vi "Init.vi"(8 "error in (no error)":errorcluster, 10 "IConfigure":refnum<class "IConfigure.lvclass">, 11 "Camera Imaqdx in":refnum<class "Camera Imaqdx.lvclass">=refnum) -> (0 "error out":errorcluster, 3 "Camera Imaqdx out":refnum<class "Camera Imaqdx.lvclass">)   [LabVIEW 2023]
uses:
  Configuration/Camera Imaqdx CFG.lvclass
  Interfaces/IConfigure/IConfigure.lvclass
  Camera Imaqdx.lvclass
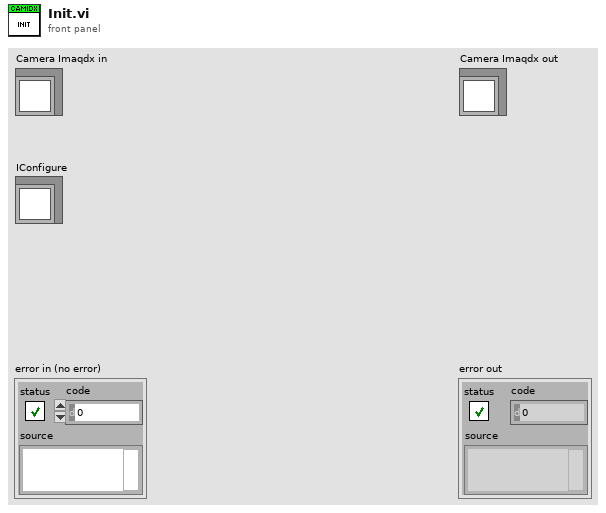
[diagram p1: front panel]
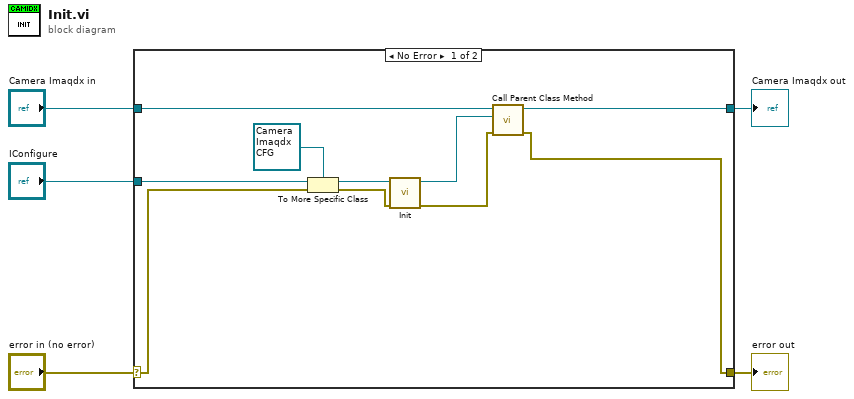
[diagram p0: block diagram]
diagram:
  n1 = case shown="No Error" "error in (no error)" {
    selector: "error in (no error)" -> [w6 w17]
    tunnel: [w8 w17] -> w4
    tunnel: [w12 w16] -> w2
    tunnel: "Camera Imaqdx in" -> [w7 w16]
    tunnel: "IConfigure" -> [w11 _]
    frame No Error {
      n2 = To More Specific Class(target class=refnum<class "Camera Imaqdx CFG.lvclass"> refnum ("Cameras.lvlib:Camera Config Imaqdx.lvclass"), reference=w11, error in=w6) -> (specific class reference=w14:refnum<class "Camera Imaqdx CFG.lvclass">, error out=w13:errorcluster)
      n3 = call-dynamic "Init.vi"("error in"=w13, "Camera Config Imaqdx in"=w14) -> ("error out"=w10:errorcluster, "Camera Config Imaqdx out"=w9:refnum<class "Camera Imaqdx CFG.lvclass">)  [unwired: 8 in]
      n4 = call-parent "Call Parent Class Method"("error in (no error)"=w10, "IConfigure"=w9, "Camera Base in"=w7) -> ("error out"=w8:errorcluster, "Camera Base out"=w12:refnum<class "Camera Imaqdx.lvclass">)  [unwired: 7 in]
    }
    frame Error {
    }
  }
  "error out" <- w4
  "Camera Imaqdx out" <- w2
